vi "type_02_int16_three_segments.vi"   [LabVIEW 2010]
types:
  T1 = enum16{"open", "open or create", "create or replace", "create", "open (read-only)"}
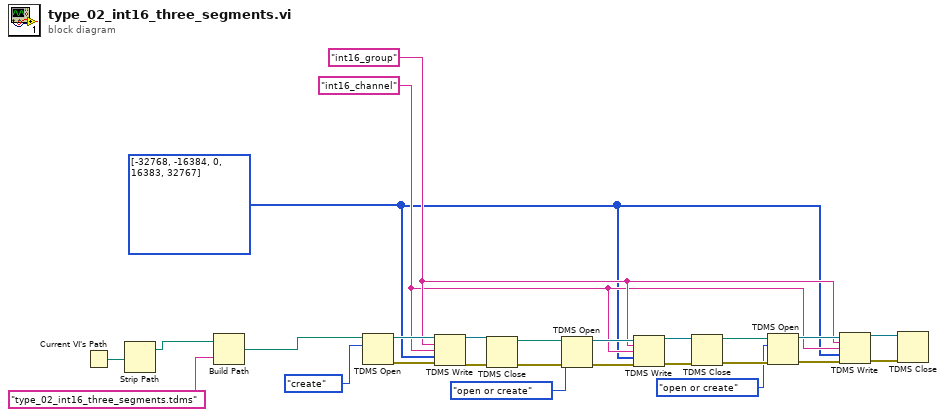
[diagram p0: block diagram]
diagram:
  w1 = i16[] [-32768, -16384, 0, 16383, 32767]
  w2 = "int16_channel" ("channel name(s) in (Untitled)")
  w3 = "int16_group" ("group name in (Untitled)")
  n1 = Current VI's Path() -> (path=w25:path)
  n2 = Strip Path(path=w25) -> (stripped path=w24:path)  [unwired: 1 out]
  n3 = Build Path(base path=w24, name or relative path="type_02_int16_three_segments.tdms") -> (appended path=w22:path)
  n4 = TDMS Open(10:T1."create" ("operation (0:open)"), 11:w22) -> (0:w12:errorcluster, 3:w11:refnum<k34>)  [unwired: 4 in]
  n5 = TDMS Write(0:w11, 5:w3, 7:w2, 9:w1, 11:w12) -> (4:w13:refnum<k34>, 15:w14:errorcluster)  [unwired: 1 in, 2 out]
  n6 = TDMS Close(8:w14, 11:w13) -> (0:w19:errorcluster, 3:w21:path)
  n7 = TDMS Open(8:w19, 10:T1."open or create" ("operation (0:open)"), 11:w21) -> (0:w18:errorcluster, 3:w17:refnum<k34>)  [unwired: 3 in]
  n8 = TDMS Write(0:w17, 5:w3, 7:w2, 9:w1, 11:w18) -> (4:w15:refnum<k34>, 15:w16:errorcluster)  [unwired: 1 in, 2 out]
  n9 = TDMS Close(8:w16, 11:w15) -> (0:w6:errorcluster, 3:w5:path)
  n10 = TDMS Open(8:w6, 10:T1."open or create" ("operation (0:open)"), 11:w5) -> (0:w10:errorcluster, 3:w9:refnum<k34>)  [unwired: 3 in]
  n11 = TDMS Write(0:w9, 5:w3, 7:w2, 9:w1, 11:w10) -> (4:w7:refnum<k34>, 15:w8:errorcluster)  [unwired: 1 in, 2 out]
  n12 = TDMS Close(8:w8, 11:w7) -> ()  [unwired: 2 out]
